vi "niRFUtil MT UTIL Validate Bit Stream.vi"(11 "Input Bit Stream":i8[](array[numeric])) -> (0 "error out":errorcluster, 1 "error?":bool)   [LabVIEW 2015, in "niRFUtil.lvlib"]
doc: "Verifies that the provided Bit Stream is valid based on:\n1. Must have at least 1 value\n2. Values can only be zero or one."
uses:
  niRFUtil.lvlib
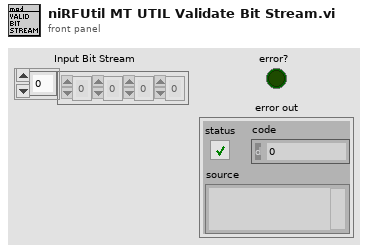
[diagram p1: front panel]
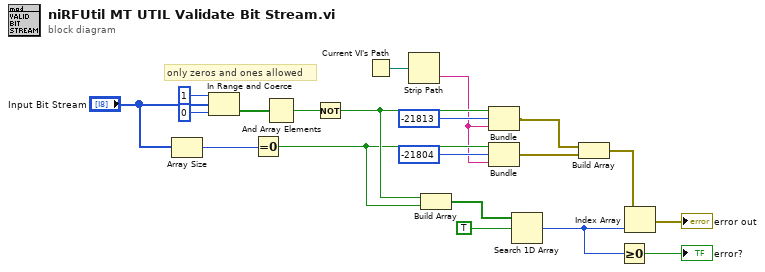
[diagram p0: block diagram]
diagram:
  # "only zeros and ones allowed"
  n1 = Array Size(array="Input Bit Stream") -> (size(s)=w6:i32)
  n2 = In Range and Coerce(upper limit=i8 1 ("Numeric"), x="Input Bit Stream", lower limit=i8 0 ("Numeric")) -> (In Range?=w13:bool[])  [unwired: 1 out]
  n3 = Equal To 0?(x=w6) -> (x = 0?=w7:bool)
  n4 = And Array Elements(Boolean array=w13) -> (logical AND=w14:bool)
  n5 = Not(x=w14) -> (.not. x?=w16:bool)
  n6 = Current VI's Path() -> (path=w20:path)
  n7 = Strip Path(path=w20) -> (name=w5:string)  [unwired: 1 out]
  n8 = Build Array(w16, w7) -> (w19:bool[])
  n9 = Bundle(w16, "code"=-21813, "name"=w5) -> (w8:cluster{bool, "code":i32, "name":string})  [unwired: 1 out]
  n10 = Bundle(w7, "code"=-21804, "name"=w5) -> (w9:cluster{bool, "code":i32, "name":string})  [unwired: 1 out]
  n11 = Search 1D Array(1D array=w19, element=TRUE) -> (index of element=w2:i32)  [unwired: 1 out]
  n12 = Build Array(w8, w9) -> (w17:cluster{bool, "code":i32, "name":string}[])
  n13 = Greater Or Equal To 0?(x=w2) -> (x >= 0?=→"error?":bool)
  n14 = Index Array(array=w17, index=w2) -> (element=→"error out":cluster{bool, "code":i32, "name":string})
